vi "Configure Remote Trace Header Filter Section.vi"(8 "error in (no error)":errorcluster, 10 "Columns (All)":i32(ring) items=["All", "Line ID", "Event Yype", "Time Stamp", "Duration", "VISA Resource", "Instrument Number", "Connection", "Data"], 11 "VISA resource name":refnum<visa-resource-name>) -> (0 "error out":errorcluster, 3 "VISA resource name out":refnum<visa-resource-name>)   [LabVIEW 2015, in "Rohde&Schwarz CMXP Base.lvlib"]
doc: "Selects which columns are shown in the trace log on the screen.\n\nAttribute:\nRSCMXPBASE_ATTR_REMOTE_TRACE_HEADER_FILTER_SECTION\n\nRemote-control command:\n[CONFigure:]BASE:RTRace:COLumns"
uses:
  <instrlib>/Rohde&Schwarz CMXP Base/Rohde&Schwarz CMXP Base.lvlib
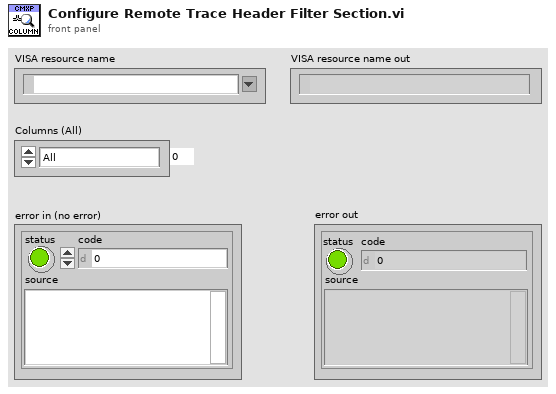
[diagram p1: front panel]
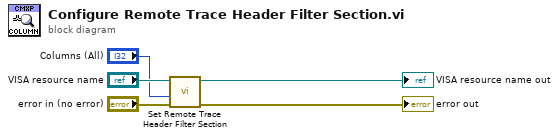
[diagram p0: block diagram]
diagram:
  n1 = call "Set Remote Trace Header Filter Section"("error in (no error)"="error in (no error)", "Remote Trace Header Filter Section (0 - All)"="Columns (All)", "instrument handle"="VISA resource name") -> ("error out"=→"error out":errorcluster, "instrument handle out"=→"VISA resource name out":refnum<visa-resource-name>)  [unwired: 7 in]
